vi "feed.vi"() -> ()   [LabVIEW 2015]
panel:
  out "feed(tforlowgoal)":bool
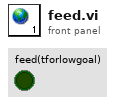
[diagram p1: front panel]
diagram:
